vi "TCP-Cllient.vi"() -> ()   [LabVIEW 2020]
doc: "演示连接TCP服务器、读取发送的数据并在图表上显示数据的方法。VI设计为TCP连接断开时停止。"
panel:
  out "波形图表 5":i32[](graph)
  out "波形图表 4":i32[][](graph)
  out "波形图表 3":i32[](graph)
  in  "file path (dialog if empty)":path caption="文件路径 （空时为对话框）"
  in  "服务器关闭":string="服务器VI关闭了连接。"
  in  "停止":bool
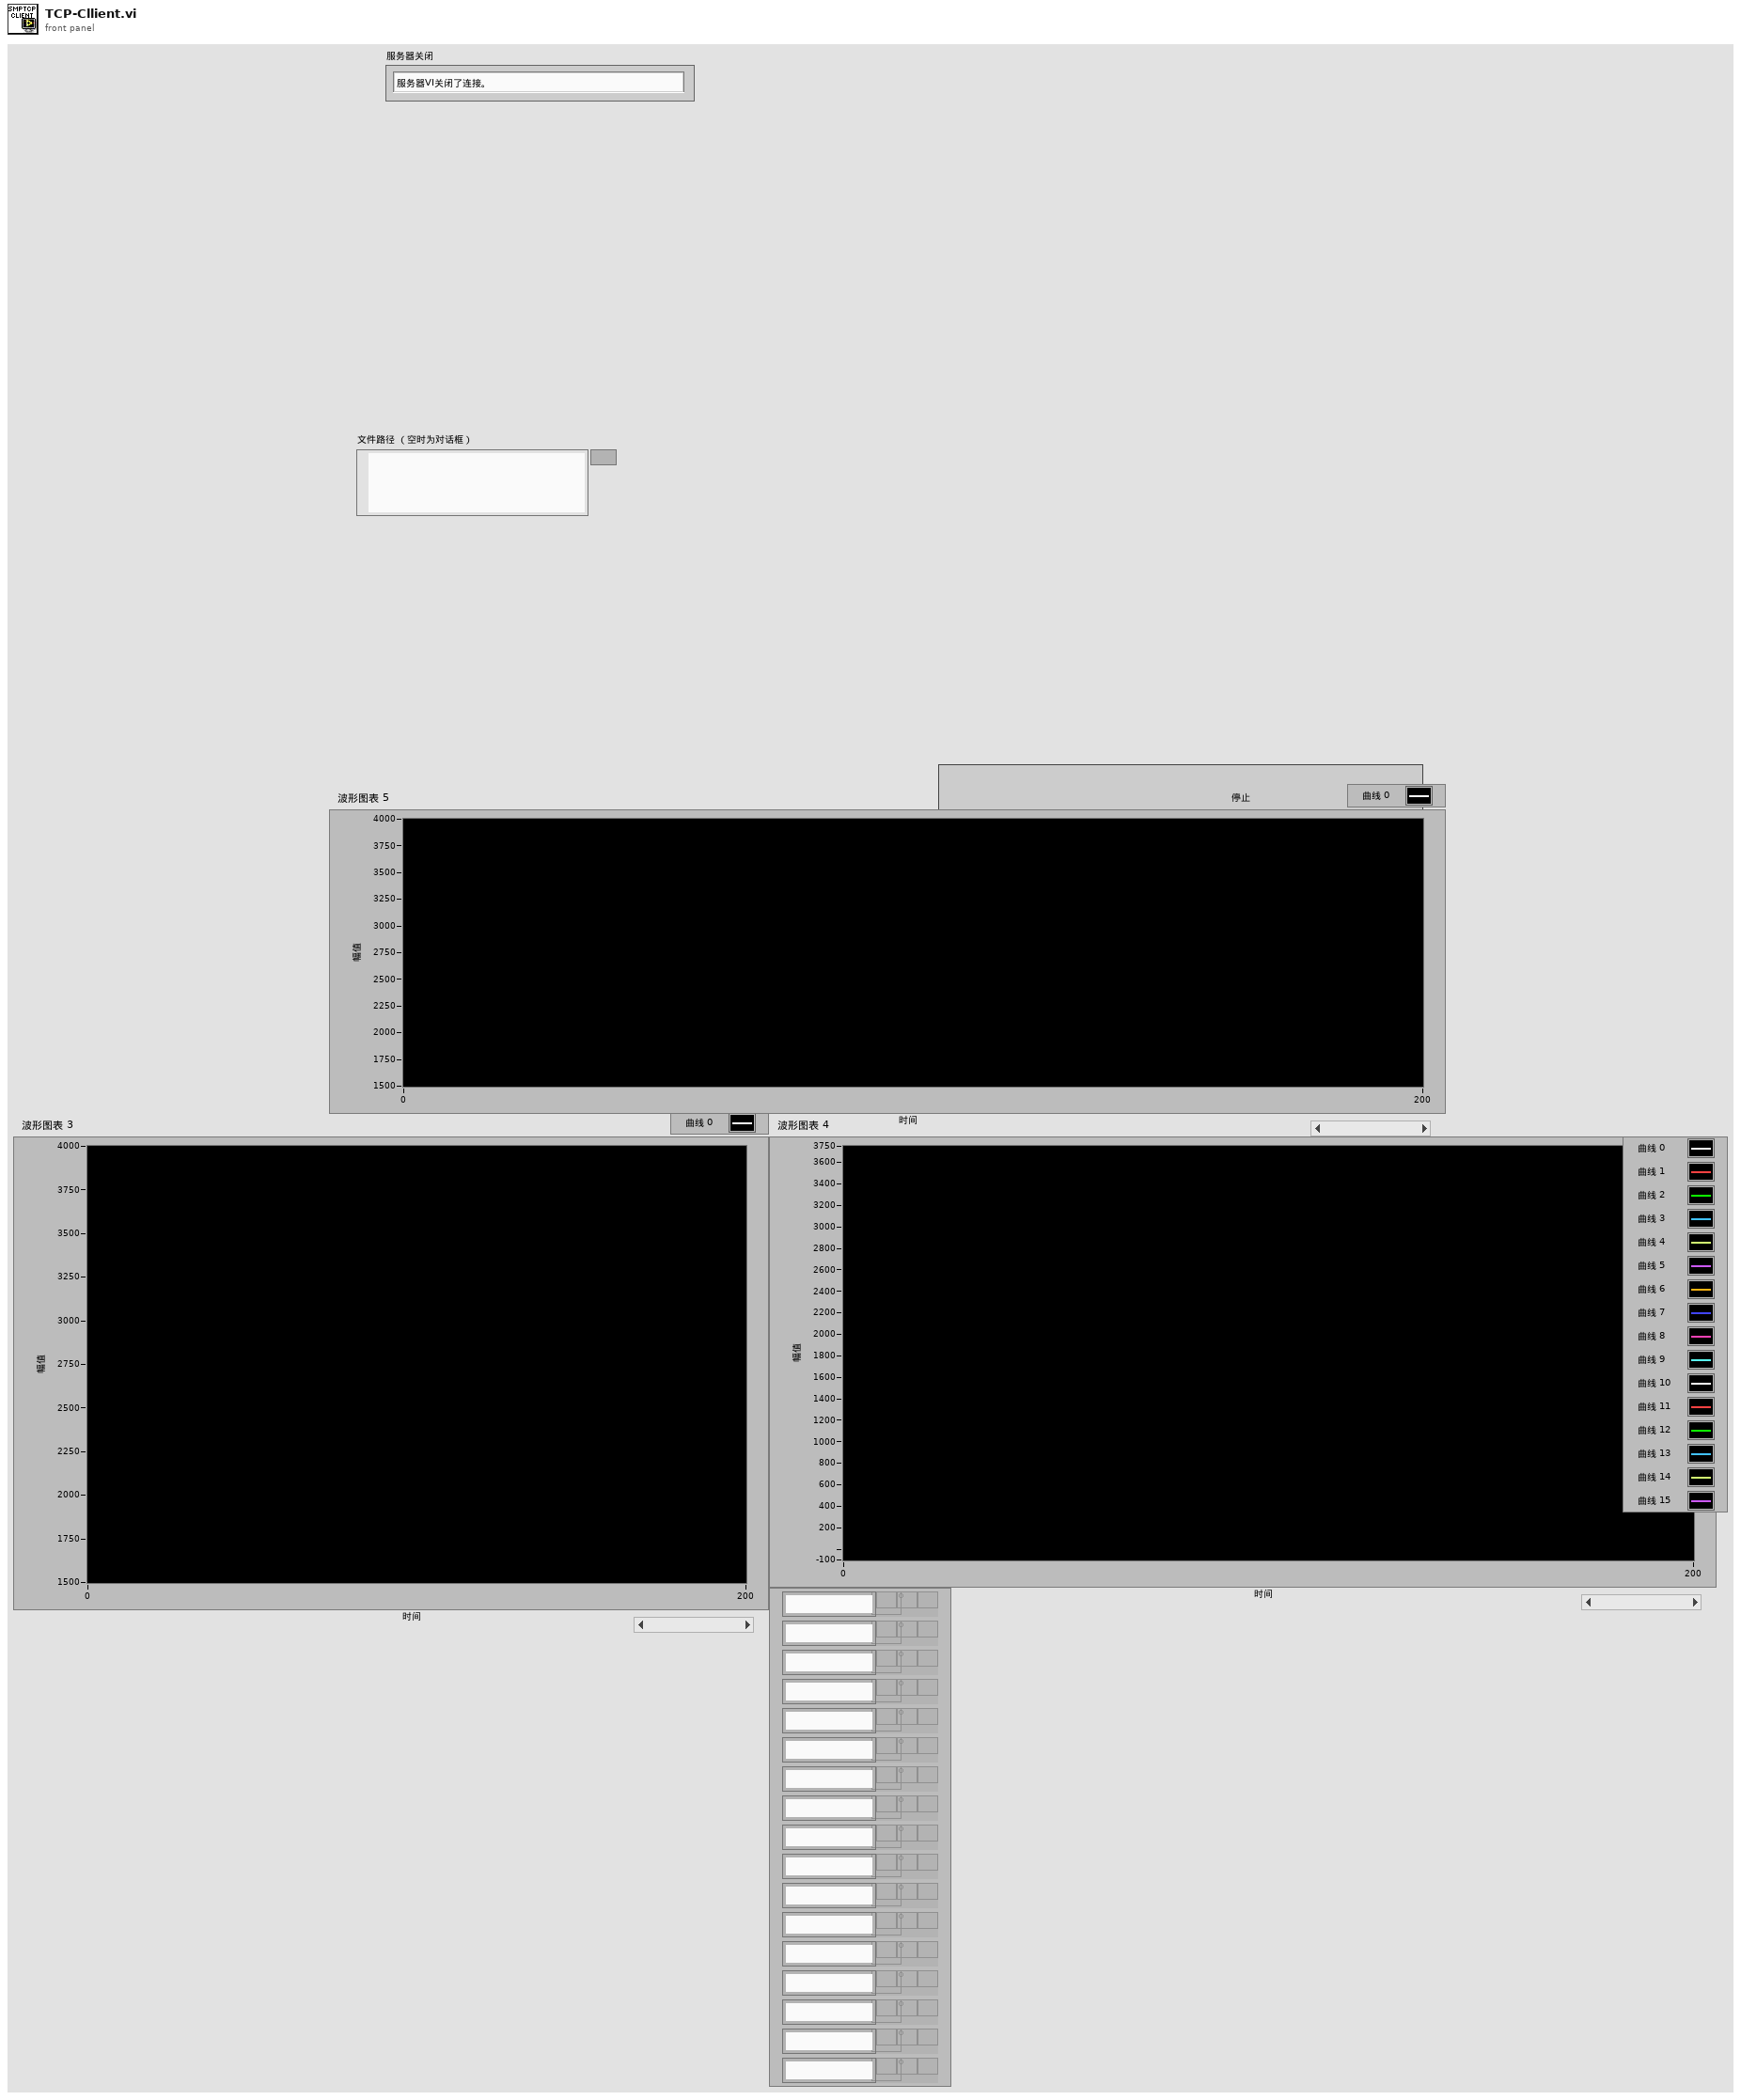
[diagram p1: front panel]
types:
  T1 = enum16{"open", "open or create", "create or replace", "create", "open (read-only)"}
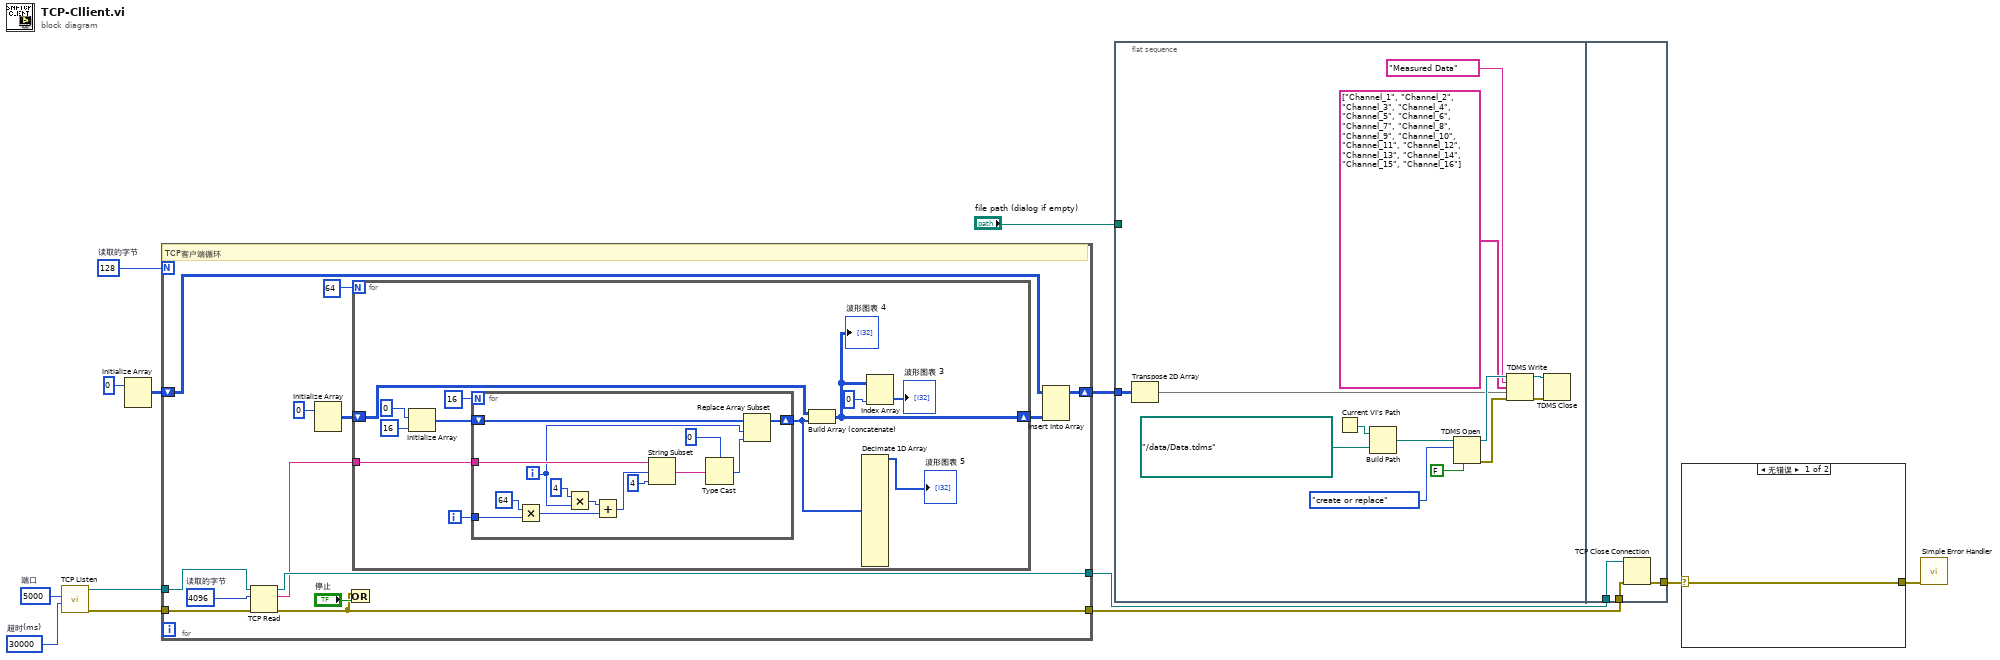
[diagram p0: block diagram]
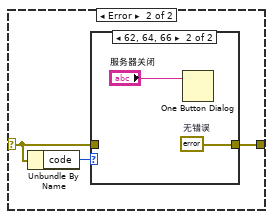
[diagram p2: hidden frame]
diagram:
  w1 = 128  # 读取的字节
  w9 = u16 5000  # 端口
  w12 = 30000  # 超时(ms)
  n1 = call <vilib>:"TCP Listen.vi"("timeout ms (wait forever: -1)"=w12, "port"=w9) -> ("error out"=w10:errorcluster, "connection ID"=w11:refnum<k5>)  [unwired: 5 in, 3 out]
  n2 = Initialize Array(0) -> (w3:i32[][])  [unwired: 2 in]
  n3 = for {
    N: w1 -> [_]
    tunnel: w10 -> [w25]
    tunnel: w11 -> [w26]
    tunnel: [w23] -> w6
    tunnel: [w22] -> w7
    shift-right: [w16] -> w2
    shift-left: w3 -> [w14]
    w21 = 4096  # 读取的字节
    # "TCP客户端循环"
    n4 = TCP Read(connection ID=w26, bytes to read=w21, error in (no error)=w25) -> (connection ID out=w23:refnum<k5>, data out=w20:string, error out=w22:errorcluster)  [unwired: 2 in]
    n5 = Initialize Array(0) -> (w17:i32[][])  [unwired: 2 in]
    n6 = Or(x=w22, y="停止") -> ()  [unwired: 1 out]
    n7 = for {
      N: u16 64 -> [_]
      tunnel: w20 -> [w38]
      shift-right: [w30] -> w15
      shift-left: w17 -> [w32]
      i -> [w33]
      n8 = Initialize Array(0, 16) -> (w34:i32[])
      n9 = for {
        N: i8 16 -> [_]
        tunnel: w38 -> [w50]
        tunnel: w33 -> [w46]
        shift-right: [w39] -> w28
        shift-left: w34 -> [w40]
        i -> [w41]
        n10 = Multiply(x=i8 64, y=w46) -> (x*y=w45:i32)
        n11 = Multiply(x=i8 4, y=w41) -> (x*y=w43:i32)
        n12 = Add(x=w43, y=w45) -> (x+y=w44:i32)
        n13 = String Subset(string=w50, offset (0)=w44, length (rest)=i8 4) -> (substring=w52:string)
        n14 = Type Cast(type=0, x=w52) -> (*(type *) &x=w42:i32)
        n15 = Replace Array Subset(array=w40, new element=w42, index=w41) -> (w39:i32[])
      }
      n16 = Build Array (concatenate)(w32, w28) -> (w30:i32[][])
      "波形图表 4" <- w30
      n17 = Decimate 1D Array(w28) -> (→"波形图表 5":i32[])  [unwired: 15 out]
      n18 = Index Array(array=w30, index (col)=0) -> (element=→"波形图表 3":i32[])  [unwired: 1 in]
    }
    n19 = Insert Into Array(array=w14, new element=w15) -> (w16:i32[][])  [unwired: 2 in]
  }
  n20 = flat-sequence {
    tunnel: "file path (dialog if empty)" -> [_]
    tunnel: w2 -> [w53]
    tunnel: w7 -> [w68]
    tunnel: w6 -> [w67]
    tunnel: [w66] -> w5
    frame #0 {
      n21 = Transpose 2D Array(2D array=w53) -> (transposed array=w55:i32[][])
      n22 = Current VI's Path() -> (path=w54:path)
      n23 = Build Path(base path=w54, name or relative path=path "../data/Data.tdms" ("file path")) -> (appended path=w61:path)
      n24 = TDMS Open(6:FALSE ("disable buffering (T)"), 10:T1."create or replace" ("operation"), 11:w61) -> (0:w65:errorcluster, 3:w62:refnum<k34>)  [unwired: 4 in]
      n25 = TDMS Write(0:w62, 5:"Measured Data" ("group name"), 7:string[] ["Channel_1", "Channel_2", "Channel_3", "Channel_4", "Channel_5", "Channel_6", "Channel_7", "Channel_8", "Channel_9", "Channel_10", "Channel_11", "Channel_12", "Channel_13", "Channel_14", "Channel_15", "Channel_16"] ("channel names"), 9:w55, 11:w65) -> (4:w63:refnum<k34>, 15:w64:errorcluster)  [unwired: 1 in, 2 out]
      n26 = TDMS Close(8:w64, 11:w63) -> ()  [unwired: 2 out]
    }
    frame #1 {
      n27 = TCP Close Connection(connection ID=w67, error in (no error)=w68) -> (error out=w66:errorcluster)  [unwired: 1 in, 1 out]
    }
  }
  n28 = case shown="无错误" w5 {
    selector: w5 -> [w69 w71]
    tunnel: [w69 w70] -> w13
    frame No Error {
    }
    frame Error {
      n29 = Unbundle By Name(w71) -> ("code"=w72:i32)
      n30 = case shown="62, 64, 66" w72 {
        tunnel: w71 -> [w73 _]
        tunnel: [w73 w75] -> w70
        frame Default {
        }
        frame 62, 64, 66 {
          w75 = errorcluster {"status"=FALSE, "code"=0, "source"=""}  # 无错误
          n31 = One Button Dialog(message="服务器关闭") -> ()  [unwired: 1 in, 1 out]
        }
      }
    }
  }
  n32 = call <vilib>:"Simple Error Handler.vi"("error in (no error)"=w13) -> ()  [unwired: 4 in, 5 out]
